vi "main.vi"() -> ()   [LabVIEW 2024]
uses:
  stateMachineStates.ctl
  statesFGV.ctl
  <vilib>/numeric/Random Number (Range) DBL.vi
panel:
  out "OutputFan":bool=TRUE
  out "temp":dbl
  in  "startTemp":dbl
  in  "stop":bool
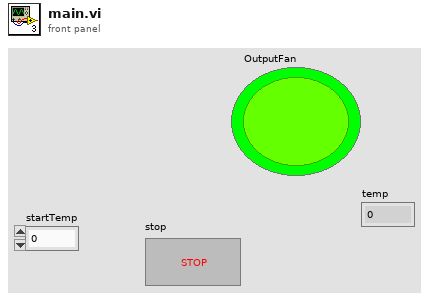
[diagram p1: front panel]
types:
  T1 = typedef "stateMachineStates.ctl" = enum16{"INIT", "IDLE", "EXIT"}
  T2 = typedef "statesFGV.ctl" = enum16{"SET", "GET"}
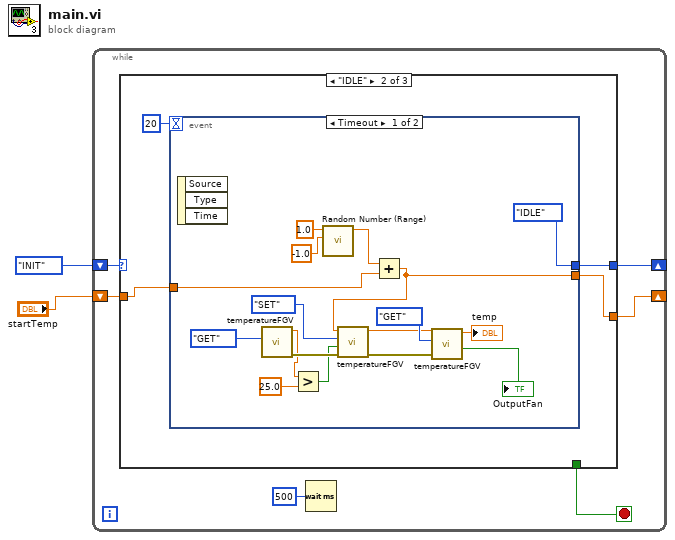
[diagram p0: block diagram]
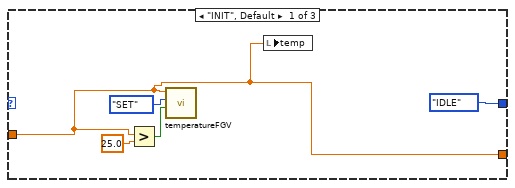
[diagram p2: hidden frame]
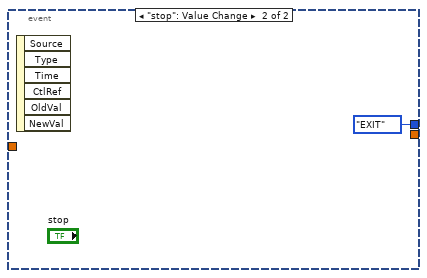
[diagram p3: hidden frame]
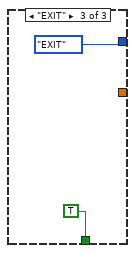
[diagram p4: hidden frame]
diagram:
  n1 = while {
    shift-right: [w5] -> _
    shift-left: stateMachineStates."INIT" -> [w8]
    shift-right: [w4] -> _
    shift-left: "startTemp" -> [w3]
    stop <- w6 stop-if-true
    n2 = case shown="\"IDLE\"" w8 {
      tunnel: [_ _ TRUE] -> w6
      tunnel: [stateMachineStates."IDLE" w17 stateMachineStates."EXIT"] -> w5
      tunnel: [w9 w15 _] -> w4
      tunnel: w3 -> [w9 w14 _]
      frame "INIT", Default {
        n3 = Greater?(x=w9, y=25.0) -> (0:w10:bool)
        n4 = call "temperatureFGV.vi"("InputFan"=w10, "state"=statesFGV."SET", "InputTemp"=w9) -> ()  [unwired: 2 in, 3 out]
        n5 = local write "temp"(w9) -> ()
      }
      frame "IDLE" {
        n6 = event shown="[0] Timeout" {
          selector: _ -> [_ _]
          dyn-events: _ -> [_ _]
          timeout: 20 -> [_ _]
          tunnel: [stateMachineStates."IDLE" stateMachineStates."EXIT"] -> w17
          tunnel: [w19 _] -> w15
          tunnel: w14 -> [w18 _]
          event Timeout {
            n7 = event-data() -> ()  [unwired: 1 in, 3 out]
            n8 = call "temperatureFGV.vi"("state"=statesFGV."GET") -> ("error out"=w31:errorcluster, "OutputTemp"=w24:dbl)  [unwired: 4 in, 1 out]
            n9 = Greater?(x=w24, y=25.0) -> (0:w22:bool)
            n10 = call-poly <vilib>:"Random Number (Range).vi"("lower bound (0)"=-1.0 ("upper bound (100)"), "upper bound (100)"=1.0) -> ("number"=w20:dbl)  [unwired: 9 in]
            n11 = Add(x=w20, y=w18) -> (x+y=w19:dbl)
            n12 = call "temperatureFGV.vi"("error in (no error)"=w31, "InputFan"=w22, "state"=statesFGV."SET", "InputTemp"=w19) -> ("error out"=w28:errorcluster, "OutputTemp"=w29:dbl)  [unwired: 1 in, 1 out]
            n13 = call "temperatureFGV.vi"("error in (no error)"=w28, "state"=statesFGV."GET", "InputTemp"=w29) -> ("OutputFan"=→"OutputFan":bool, "OutputTemp"=→"temp":dbl)  [unwired: 2 in, 1 out]
          }
          event "stop": Value Change {
            n14 = event-data() -> ()  [unwired: 1 in, 6 out]
          }
        }
      }
      frame "EXIT" {
      }
    }
    n15 = Wait (ms)(milliseconds to wait=u32 500) -> ()  [unwired: 1 out]
  }
